vi "iWorx - Polar Heart Rate Monitor.vi"() -> ()   [LabVIEW 2012]
uses:
  <vilib>/DAQmx/create/channels.llb/DAQmx Create Channel (AI-Voltage-Basic).vi
  <vilib>/DAQmx/configure/timing.llb/DAQmx Timing (Sample Clock).vi
  <vilib>/Analysis/baseanly.llb/Mean (DBL).vi
  <vilib>/DAQmx/read.llb/DAQmx Read (Analog 1D Wfm NChan NSamp).vi
  <vilib>/measure/macond.llb/IIR Filter for 1 Chan.vi
  <vilib>/measure/NI_MAPro.lvlib
  <vilib>/Analysis/NI_AALBase.lvlib
panel:
  in  "Stop":bool
  in  "Reset Scale":bool
  in  "Log Info Button":bool
  out "error out":errorcluster
  out "Inst Pulse Rate":dbl format="%5.1f BPM"
  out "Avg Pulse Rate":dbl format="%5.1f BPM"
  in  "Calibrate":bool
  in  "Set Up":bool
  out "Waveform Chart":waveform(dbl)(graph)={"t0"=timestamp(3473276322.092825 s since 1904-01-01), "dt"=9.999999999999999e-05, "Y"=array[2001 elements], "attributes"=variant("NI_ChannelName"=variant(string "myDAQ1/audioInputLeft"), "NI_UnitDescription"=variant(string "Volts"))}
  in  "Threashold":dbl=0.08 format="%#_g V"
  in  "Channel":u16(ring) items=["Channel 1", "Channel 2"]
  in  "Pause Button":bool
  in  "Snapshot":bool
  in  "Clear Chart":bool
  in  "Open Log":bool
  in  "Rescale Y":bool
  out "Raw Signal":dbl(knob) scale=-1.0..1.0
  # "iWorx - Polar Heart Rate Monitor - Data Logger"
  # "Sensor Input"
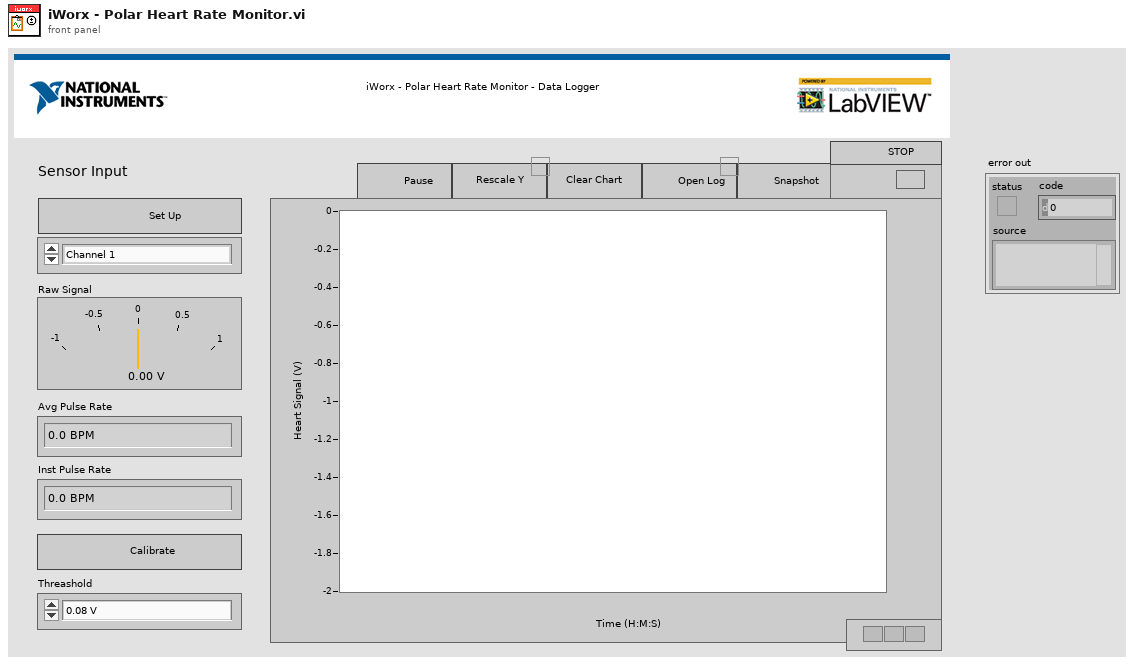
[diagram p1: front panel]
types:
  T1 = cluster{"Topology":enum16{"Off", "Butterworth", "Chebyshev", "Inverse Chebyshev", "Elliptic", "Bessel"}, "Type":enum16{"Lowpass", "Highpass", "Bandpass", "Bandstop"}, "Order":i32, "Lower Fc":dbl, "Upper Fc":dbl, "PB Ripple":dbl, "SB Attenuation":dbl}
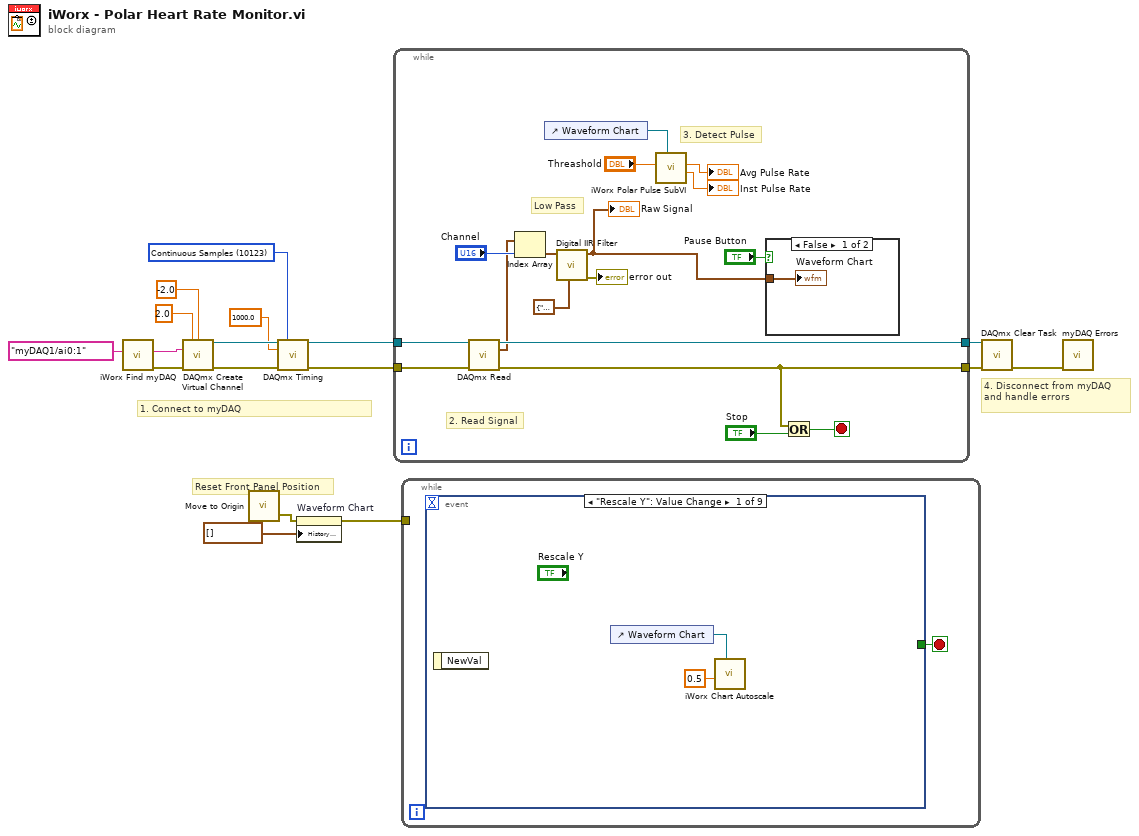
[diagram p0: block diagram]
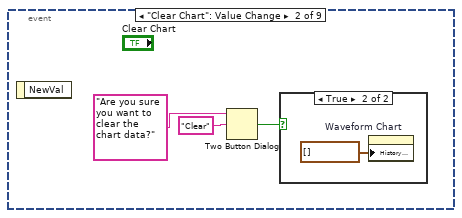
[diagram p2: hidden frame]
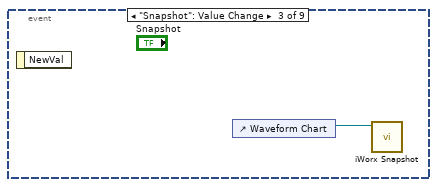
[diagram p4: hidden frame]
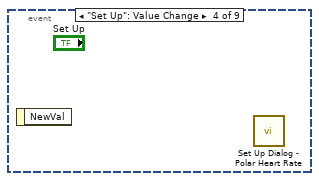
[diagram p5: hidden frame]
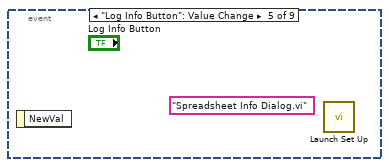
[diagram p6: hidden frame]
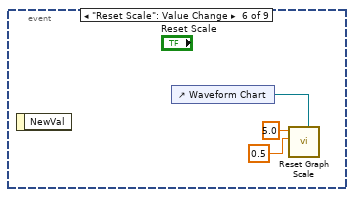
[diagram p7: hidden frame]
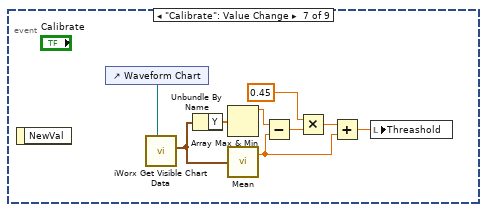
[diagram p8: hidden frame]
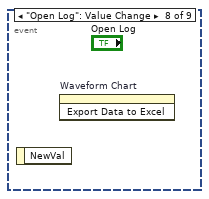
[diagram p9: hidden frame]
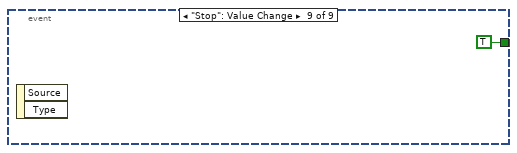
[diagram p10: hidden frame]
diagram:
  w9 = 10123 items=["Finite Samples"=10178, "Continuous Samples"=10123, "Hardware Timed Single Point"=12522] ("sample mode")
  # "1. Connect to myDAQ"
  # "Reset Front Panel Position"
  # "4. Disconnect from myDAQ and handle errors"
  n1 = call "iWorx Find myDAQ.vi"("Preferred myDAQ (myDAQ1)"=tag "myDAQ1/ai0:1" ("physical channels")) -> ("Error Out"=w5:errorcluster, "DAQmx Physical Channel"=w4:tag)  [unwired: 6 in, 3 out]
  n2 = call-poly <vilib>:"DAQmx Create Virtual Channel.vi"("maximum value"=2.0, "minimum value"=-2.0, "physical channels"=w4, "error in"=w5) -> ("task out"=w13:refnum<k21>, "error out"=w12:errorcluster)  [unwired: 10 in]
  n3 = call "Move to Origin.vi"() -> ("Error Out"=w1:errorcluster)  [unwired: 3 in]
  n4 = call-poly <vilib>:"DAQmx Timing.vi"("task/channels in"=w13, "sample mode"=w9, "rate"=1000.0, "error in"=w12) -> ("task out"=w10:refnum<k21>, "error out"=w11:errorcluster)  [unwired: 10 in]
  n5 = property on="Waveform Chart" class="WFChart (strict)"(error in=w1, "History Data"=waveform(dbl)[] []) -> (error out=w15:errorcluster)  [unwired: 1 in, 1 out]
  n6 = while {
    tunnel: w10 -> [w34]
    tunnel: [w33] -> w17
    tunnel: w11 -> [w32]
    tunnel: [w28] -> w16
    stop <- w31 stop-if-true
    # "3. Detect Pulse"
    # "2. Read Signal"
    # "Low Pass"
    n7 = call-poly <vilib>:"DAQmx Read.vi"("task/channels in"=w34, "error in"=w32) -> ("task out"=w33:refnum<k21>, "data"=w27:waveform(dbl)[], "error out"=w28:errorcluster)  [unwired: 11 in]
    n8 = Index Array(array=w27, index="Channel") -> (element=w26:waveform(dbl))
    n9 = control-ref of="Waveform Chart"() -> (w24:refnum<vi>)
    n10 = call-poly <vilib>:"Digital IIR Filter.vi"("IIR filter specifications"=T1 {"Topology"=enum."Butterworth", "Type"=enum."Lowpass", "Order"=2, "Lower Fc"=20.0, "Upper Fc"=200.0, "PB Ripple"=1.0, "SB Attenuation"=60.0}, "signal in"=w26) -> ("error out"=→"error out":errorcluster, "signal out"=w19:waveform(dbl))  [unwired: 7 in, 1 out]
    "Raw Signal" <- w19
    n11 = call "iWorx Polar Pulse SubVI.vi"("Waveform Chart Ref"=w24, "Threashold"="Threashold") -> ("Inst Pulse Rate"=→"Inst Pulse Rate":dbl, "Avg Pulse Rate"=→"Avg Pulse Rate":dbl)  [unwired: 7 in, 1 out]
    n12 = case shown="False" "Pause Button" {
      tunnel: w19 -> [w35 _]
      frame False {
        "Waveform Chart" <- w35
      }
      frame True {
      }
    }
    n13 = Or(x=w28, y="Stop") -> (x .or. y?=w31:bool)
  }
  n14 = while {
    tunnel: w15 -> [_]
    stop <- w36 stop-if-true
    n15 = event shown="[0] \"Rescale Y\": Value Change" {
      selector: _ -> [_ _ _ _ _ _ _ _ _]
      dyn-events: _ -> [_ _ _ _ _ _ _ _ _]
      timeout: _ -> [_ _ _ _ _ _ _ _ _]
      tunnel: [_ _ _ _ _ _ _ _ TRUE] -> w36
      event "Rescale Y": Value Change {
        n16 = event-data() -> ()  [unwired: 1 in, 1 out]
        n17 = control-ref of="Waveform Chart"() -> (w37:refnum<vi>)
        n18 = call "iWorx Chart Autoscale.vi"("Selection Chart"=w37, "Rounding Multiple (10)"=0.5 ("Rounding Multiple (1)")) -> ()  [unwired: 7 in, 3 out]
      }
      event "Clear Chart": Value Change {
        n19 = event-data() -> ()  [unwired: 1 in, 1 out]
        n20 = Two Button Dialog(message="Are you sure you want to clear the chart data?", 2:"Clear" ("T button name (\"OK\")")) -> (T button?=w40:bool)  [unwired: 1 in]
        n21 = case shown="True" w40 {
          frame False {
          }
          frame True {
            n22 = property on="Waveform Chart" class="WFChart (strict)"("History Data"=waveform(dbl)[] []) -> ()  [unwired: 2 in, 2 out]
          }
        }
      }
      event "Snapshot": Value Change {
        n23 = event-data() -> ()  [unwired: 1 in, 1 out]
        n24 = control-ref of="Waveform Chart"() -> (w43:refnum<vi>)
        n25 = call "iWorx Snapshot.vi"("WaveformChart in"=w43) -> ()  [unwired: 10 in, 1 out]
      }
      event "Set Up": Value Change {
        n26 = event-data() -> ()  [unwired: 1 in, 1 out]
        n27 = call "Set Up Dialog - Polar Heart Rate.vi"() -> ()  [unwired: 12 in]
      }
      event "Log Info Button": Value Change {
        (unwired) "Spreadsheet Info Dialog.vi" ("name or relative path")
        n28 = event-data() -> ()  [unwired: 1 in, 1 out]
        n29 = call "Launch Set Up.vi"() -> ()  [unwired: 10 in, 2 out]
      }
      event "Reset Scale": Value Change {
        n30 = event-data() -> ()  [unwired: 1 in, 1 out]
        n31 = control-ref of="Waveform Chart"() -> (w44:refnum<vi>)
        n32 = call "Reset Graph Scale.vi"("WaveformChart in"=w44, "Minimum (0)"=0.5 ("Maximum (100)"), "Maximum (100)"=5.0) -> ()  [unwired: 8 in, 1 out]
      }
      event "Calibrate": Value Change {
        n33 = event-data() -> ()  [unwired: 1 in, 1 out]
        n34 = control-ref of="Waveform Chart"() -> (w55:refnum<vi>)
        n35 = call "iWorx Get Visible Chart Data.vi"("Selection Chart"=w55) -> ("waveform out"=w54:waveform(dbl))  [unwired: 8 in, 2 out]
        n36 = Unbundle By Name(w54) -> ("Y"=w53:dbl[])
        n37 = Array Max & Min(array=w53) -> (max value=w52:dbl)  [unwired: 3 out]
        n38 = call-poly <vilib>:"Mean.vi"("X"=w54) -> ("mean"=w48:dbl)  [unwired: 1 out]
        n39 = Subtract(x=w52, y=w48) -> (x-y=w51:dbl)
        n40 = Multiply(x=0.45, y=w51) -> (x*y=w49:dbl)
        n41 = Add(x=w49, y=w48) -> (x+y=w47:dbl)
        n42 = local write "Threashold"(w47) -> ()
      }
      event "Open Log": Value Change {
        n43 = event-data() -> ()  [unwired: 1 in, 1 out]
        n44 = invoke on="Waveform Chart" class="WFChart (strict)" method="Export Data to Excel"() -> ()  [unwired: 3 in, 3 out]
      }
      event "Stop": Value Change {
        n45 = event-data() -> ()  [unwired: 1 in, 2 out]
      }
    }
  }
  n46 = call <vilib>:"DAQmx Clear Task.vi"("task in"=w17, "error in"=w16) -> ("error out"=w2:errorcluster)  [unwired: 13 in]
  n47 = call "myDAQ Errors.vi"("error in (no error)"=w2) -> ()  [unwired: 10 in, 1 out]
